vi "Convert_GroupOfDTCs.vi"(1 "group of DTC":u32, 2 "DTC descriptor":T1={"DTC Byte Length"=2, "Status Byte Length"=1, "Add Data Byte Length"=0, "Byte Order"=enum."Motorola"}) -> (0 "data out":u8[](array[numeric]))   [LabVIEW 2014]
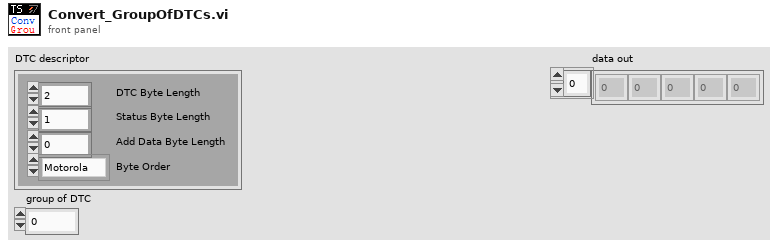
[diagram p1: front panel]
types:
  T1 = cluster{"DTC Byte Length":i32, "Status Byte Length":i32, "Add Data Byte Length":i32, "Byte Order":enum16{"Motorola", "Intel"}}
  T2 = cluster{"Start Byte":i32, "Byte Length":i32, "Byte Order":enum16{"Motorola", "Intel"}, "Data Type":enum16{"Unsigned", "Signed", "Float"}, "Scale Factor":dbl, "Scale Offset":dbl}
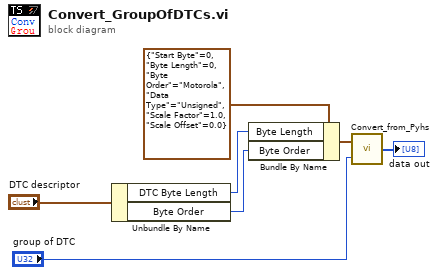
[diagram p0: block diagram]
diagram:
  n1 = Unbundle By Name("DTC descriptor") -> ("DTC Byte Length"=w3:i32, "Byte Order"=w4:enum16{"Motorola", "Intel"})
  n2 = Bundle By Name(cluster=T2 {"Start Byte"=0, "Byte Length"=0, "Byte Order"=enum."Motorola", "Data Type"=enum."Unsigned", "Scale Factor"=1.0, "Scale Offset"=0.0} ("type descriptor"), "Byte Length"=w3, "Byte Order"=w4) -> (w5:T2)
  n3 = call "Convert_from_Pyhs.vi"("group of DTC"="group of DTC", "type descriptor"=w5) -> ("data out"=→"data out":u8[])
